vi "manual_comparison.vi"(8 "error in (no error)":errorcluster, 11 "data":variant) -> (0 "error out":errorcluster)   [LabVIEW 2015, in "lv-recipe-machine.lvlib" / "example_01.lvlib"]
doc: "manual_comparison.vi will generate a random number between 1 and 2000 and compare to the provided value or if no value (double) is provided it will generate a random number between 1 and 2000. IT's output will provide a boolean if the random number is greater than or equal to the comparison value."
uses:
  example_01.lvlib
  _controls/steps_actions_data.ctl
  _controls/steps_actions.ctl
  lv-recipe-machine.lvlib
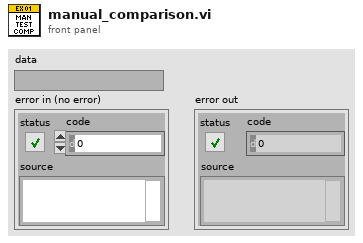
[diagram p1: front panel]
types:
  T1 = typedef "lv-recipe-machine.lvlib/example_01.lvlib/steps_actions.ctl" = enum16{"<steps_actions>", "manual_random", "manual_comparison", "manual_wait", "auto_random", "auto_wait", "criteria_initialize", "criteria_count", "criteria_comparison", "transition_simple", "transition_count", "transition_comparison", "launch_wait", "<null>"}
  T2 = typedef "lv-recipe-machine.lvlib/example_01.lvlib/steps_actions_data.ctl" = cluster{"step_action":T1, "data":variant}
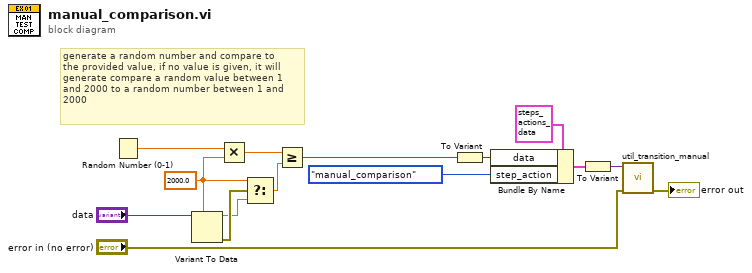
[diagram p0: block diagram]
diagram:
  w1 = 2000.0
  # "generate a random number and compare to\nthe provided value, if no value is given, it will\ngenerate compare a random value between 1\nand 2000 to a random number between 1 and\n2000"
  n1 = Random Number (0-1)() -> (number: 0 to 1=w3:dbl)
  n2 = Variant To Data(type=w1, Variant="data") -> (data=w10:dbl, error out=w11:errorcluster)  [unwired: 1 in]
  n3 = Multiply(x=w3, y=w1) -> (x*y=w2:dbl)
  n4 = Select(t=w1, s=w11, f=w10) -> (s? t:f=w4:dbl)
  n5 = Greater Or Equal?(x=w2, y=w4) -> (x >= y?=w9:bool)
  n6 = To Variant(anything=w9) -> (Variant=w13:variant)
  n7 = Bundle By Name(cluster=T2 {"step_action"=enum."<steps_actions>", "data"=variant}, "data"=w13, "step_action"=steps_actions."manual_comparison" ("manual_action")) -> (w8:T2)
  n8 = To Variant(anything=w8) -> (Variant=w7:variant)
  n9 = call "util_transition_manual.vi"("error in (no error)"="error in (no error)", "data"=w7) -> ("error out"=→"error out":errorcluster)  [unwired: 9 in]
